vi "To and From String Array.vi"() -> (0 "error out":errorcluster, 2 "Pass":bool)   [LabVIEW 2014, in "Scan Engine tests.lvlib"]
uses:
  Scan Engine tests.lvlib
  configuration/Scan Engine configuration.lvclass/Scan Engine configuration.ctl
  <vilib>/NI/Tag Bus Module Framework/channel/TBM channel.lvclass
  configuration/Scan Engine configuration.lvclass
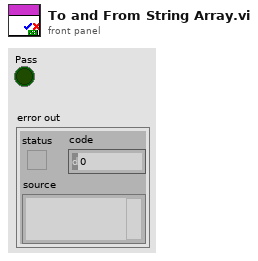
[diagram p1: front panel]
types:
  T1 = typedef "Scan Engine configuration.lvclass/Line.ctl" = cluster{"channel":refnum<class "TBM channel.lvclass">, "Tag":string}
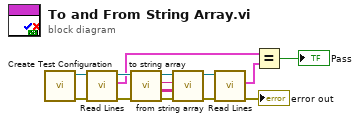
[diagram p0: block diagram]
diagram:
  n1 = call "Create Test Configuration.vi"() -> ("error out"=w9:errorcluster, "module"=w12:refnum<class "Scan Engine configuration.lvclass">)  [unwired: 6 in, 4 out]
  n2 = call "Read Lines.vi"("error in (no error)"=w9, "Scan Engine configuration in"=w12) -> ("error out"=w8:errorcluster, "Lines"=w4:T1[], "Scan Engine configuration out"=w11:refnum<class "Scan Engine configuration.lvclass">)  [unwired: 7 in]
  n3 = call-dynamic "to string array.vi"("error in (no error)"=w8, "module configuration in"=w11) -> ("error out"=w7:errorcluster, "Array"=w13:string[][], "version"=w14:string, "module configuration out"=w1:refnum<class "Scan Engine configuration.lvclass">)  [unwired: 6 in]
  n4 = call-dynamic "from string array.vi"("error in (no error)"=w7, "String Array"=w13, "version"=w14, "module configuration in"=w1) -> ("error out"=w6:errorcluster, "module configuration out"=w10:refnum<class "Scan Engine configuration.lvclass">)  [unwired: 6 in]
  n5 = call "Read Lines.vi"("error in (no error)"=w6, "Scan Engine configuration in"=w10) -> ("error out"=→"error out":errorcluster, "Lines"=w3:T1[])  [unwired: 7 in, 1 out]
  n6 = Equal?(x=w4, y=w3) -> (x = y?=→"Pass":bool)
